vi "Configure.vi"(8 "error in (no error)":errorcluster, 10 "Configuration":refnum<class "Column Configuration.lvclass">, 11 "Basic Column Factory in":refnum<class "Basic Column Factory.lvclass">) -> (0 "error out":errorcluster, 3 "Basic Column Factory out":refnum<class "Basic Column Factory.lvclass">)   [LabVIEW 2020, in "Basic Columns.lvlib" / "Basic Column Factory.lvclass"]
uses:
  Basic Column Factory.lvclass
  Basic Column Configuration Class/Column Configuration.lvclass
  Basic Column Factory.lvclass/Basic Column Factory.ctl
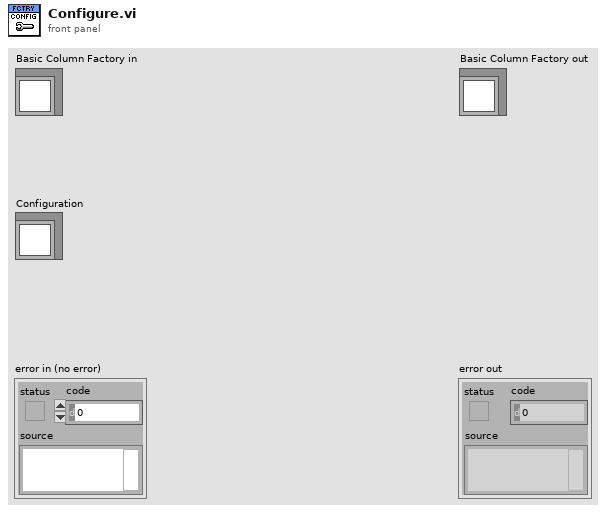
[diagram p1: front panel]
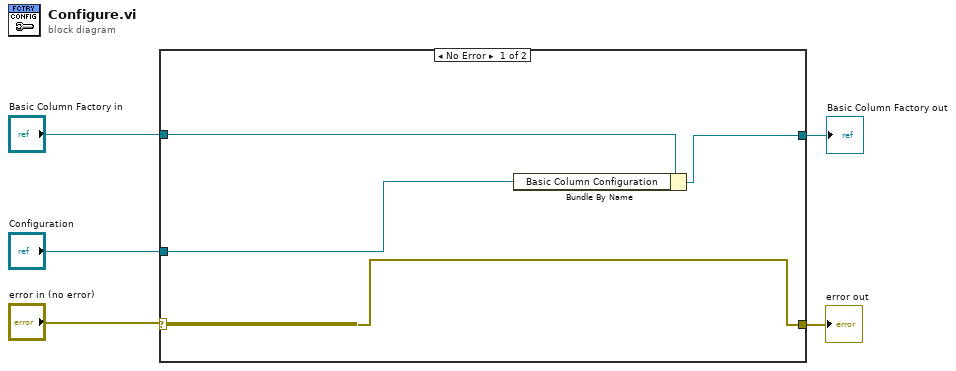
[diagram p0: block diagram]
diagram:
  n1 = case shown="No Error" "error in (no error)" {
    selector: "error in (no error)" -> [w6 w11]
    tunnel: [w6 w11] -> w2
    tunnel: "Basic Column Factory in" -> [w9 w10]
    tunnel: "Configuration" -> [w7 _]
    tunnel: [w8 w10] -> w1
    frame No Error {
      n2 = Bundle By Name(cluster=w9, "Basic Column Configuration"=w7) -> (w8:refnum<class "Basic Column Factory.lvclass">)
    }
    frame Error {
    }
  }
  "error out" <- w2
  "Basic Column Factory out" <- w1
